vi "CAN Example.vi"() -> ()   [LabVIEW 2019]
uses:
  <vilib>/xnet/xnet.llb/XNET Create Session (Frame Input Stream).vi
  Wrapper API/support/Create CANBus Load Calculator.vi
  <vilib>/xnet/xnet.llb/XNET Read (Frame CAN).vi
  Wrapper API/support/Add CANBus Received Frames.vi
  XNET-Bus-Load-Calculator.lvlib
  <resource>/objmgr/xnet.rc
panel:
  out "Bus Load (%)":dbl(graph)
  in  "stop":bool
  in  "Calculation Period (ms)":u32=500
  in  "cluster (:memory:)":refnum<k21>="BusLoad_DB"
  in  "CAN Interface":refnum<k21>="CAN1"
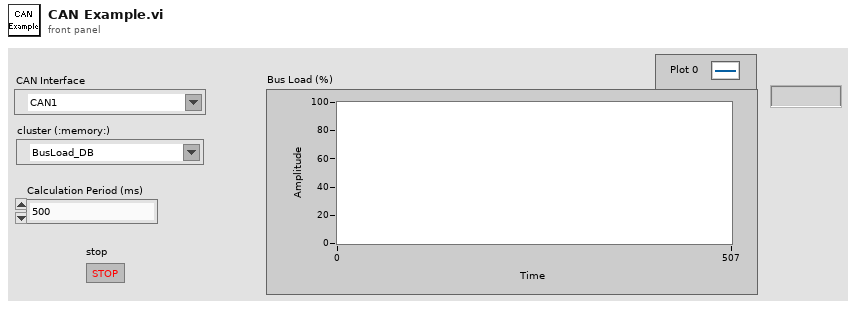
[diagram p1: front panel]
types:
  T1 = typedef "XNET Frame CAN.ctl" = cluster{"timestamp":timestamp, "payload":u8[], "identifier":u32, "type":T2, "extended?":bool, "echo?":bool}
  T2 = typedef "XNET Frame Type CAN.ctl" = u8
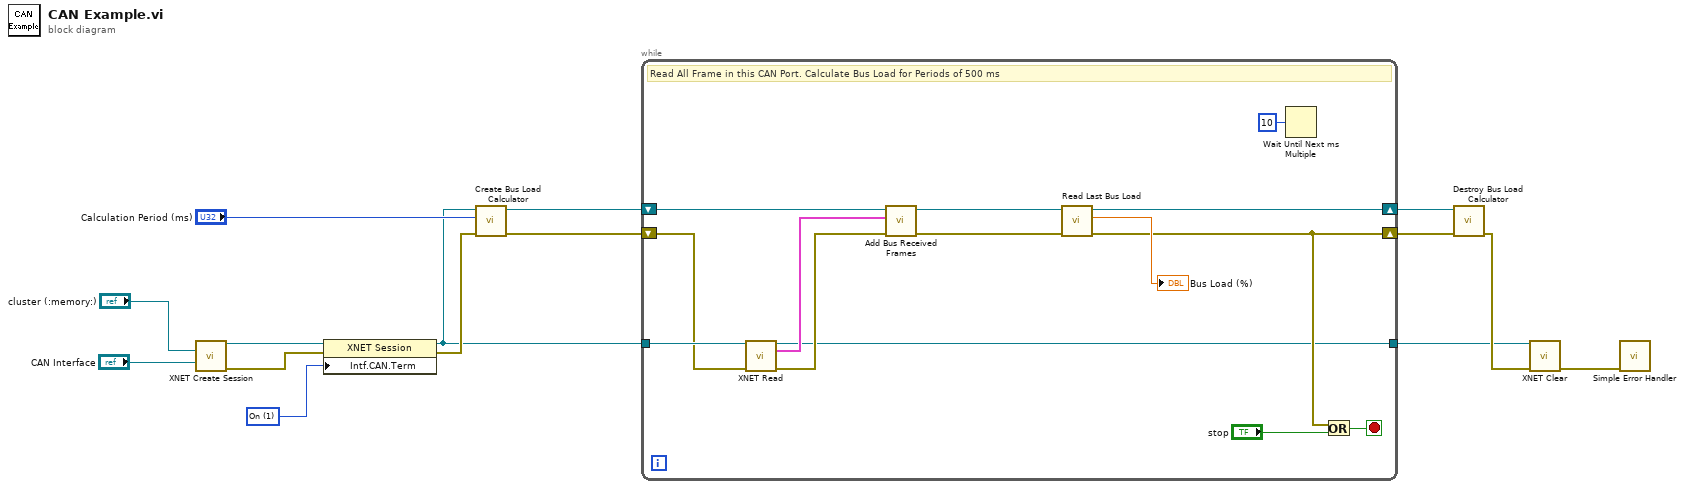
[diagram p0: block diagram]
diagram:
  w1 = u32 1 items=["Off", "On"] ("Interface:CAN:Termination")
  n1 = call-poly <vilib>:"XNET Create Session.vi"("cluster (:memory:)"="cluster (:memory:)", "interface"="CAN Interface") -> ("session out"=w3:refnum<k21>, "error out"=w14:errorcluster)  [unwired: 12 in]
  n2 = property class="XNET Session"(reference=w3, error in=w14, "Intf.CAN.Term"=w1) -> (reference out=w2:refnum<k21>, error out=w4:errorcluster)
  n3 = call-poly "Create Bus Load Calculator.vi"("error in (no error)"=w4, "Calculation Period (ms)"="Calculation Period (ms)", "XNET Session"=w2) -> ("error out"=w11:errorcluster, "Load Calculator"=w15:refnum<class "GenBus_Load_Calculator.lvclass">)  [unwired: 7 in]
  n4 = while {
    tunnel: w2 -> [w28]
    shift-right: [w22] -> w9
    shift-left: w15 -> [w29]
    shift-right: [w17] -> w8
    shift-left: w11 -> [w27]
    tunnel: [w16] -> w6
    stop <- w21 stop-if-true
    # "Read All Frame in this CAN Port. Calculate Bus Load for Periods of 500 ms"
    n5 = call-poly <vilib>:"XNET Read.vi"("session in"=w28, "error in (no error)"=w27) -> ("session out"=w16:refnum<k21>, "data"=w26:T1[], "error out"=w20:errorcluster)  [unwired: 10 in, 1 out]
    n6 = call-poly "Add Bus Received Frames.vi"("error in (no error)"=w20, "CAN Frames"=w26, "Load Calculator in"=w29) -> ("error out"=w23:errorcluster, "Load Calculator out"=w24:refnum<class "GenBus_Load_Calculator.lvclass">)  [unwired: 7 in]
    n7 = call "Read Last Bus Load.vi"("error in (no error)"=w23, "Load Calculator in"=w24) -> ("error out"=w17:errorcluster, "Bus Load (%)"=→"Bus Load (%)":dbl, "Load Calculator out"=w22:refnum<class "GenBus_Load_Calculator.lvclass">)  [unwired: 7 in]
    n8 = Wait Until Next ms Multiple(millisecond multiple=u32 10) -> ()  [unwired: 1 out]
    n9 = Or(x=w17, y="stop") -> (x .or. y?=w21:bool)
  }
  n10 = call "Destroy Bus Load Calculator.vi"("error in (no error)"=w8, "Load Calculator"=w9) -> ("error out"=w7:errorcluster)  [unwired: 9 in]
  n11 = call <vilib>:"XNET Clear.vi"("session in"=w6, "error in (no error)"=w7) -> ("error out"=w5:errorcluster)  [unwired: 13 in]
  n12 = call <vilib>:"Simple Error Handler.vi"("error in (no error)"=w5) -> ()  [unwired: 4 in, 5 out]
